vi "P4CMD Get File Copy.vi"(6 "version":string, 8 "error in (no error)":errorcluster, 9 "target filename":path, 10 "source filename":path, 11 "source control reference in":T1) -> (0 "error out":errorcluster, 2 "status message":string, 3 "source control reference out":T1)   [LabVIEW 2020, in "NI_SCC_P4CMD.lvlib"]
uses:
  <vilib>/SourceControl/Providers/P4CMD/NI_SCC_P4CMD.lvlib
  <vilib>/SourceControl/sccapi/SCCAPI Refnum.ctl
  <vilib>/SourceControl/Providers/P4CMD/P4CMD Operations.ctl
  <vilib>/SourceControl/support/SCCSup Message Strings GLBL.vi
  <vilib>/SourceControl/sccapi/NI_SCC.lvlib
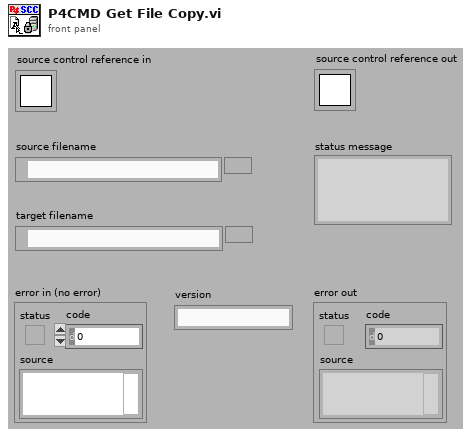
[diagram p1: front panel]
types:
  T1 = typedef "NI_SCC.lvlib/SCCAPI Refnum.ctl" = refnum<k1>
  T2 = typedef "NI_SCC_P4CMD.lvlib/P4CMD Operations.ctl" = enum16{"get all clients", "get all users", "describe changelist", "sync from depot", "open for edit", "submit to depot", "revert", "add to depot", "remove from depot", "print files revisions", "compare client file", "print depot file contents", "list opened files", "get file info", "lock files", "edit changelist spec", "info", "set variables"}
  T3 = typedef "NI_SCC_P4CMD.lvlib/P4CMD SCC File Status.ctl" = cluster{"source controlled":bool, "open by user":bool, "open by other":bool, "out of date":bool, "deleted":bool, "locked by user":bool, "locked by other":bool, "open for add by user":bool, "open for delete by user":bool}
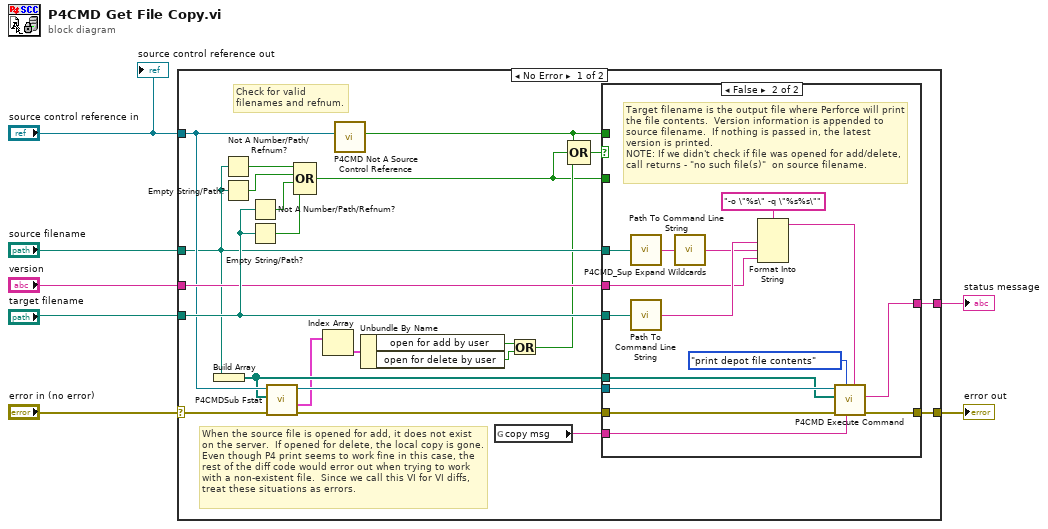
[diagram p0: block diagram]
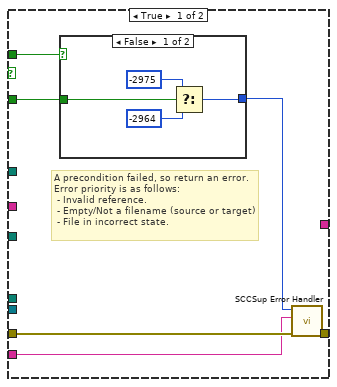
[diagram p2: hidden frame]
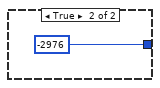
[diagram p3: hidden frame]
diagram:
  n1 = case shown="No Error" "error in (no error)" {
    selector: "error in (no error)" -> [w19 w57]
    tunnel: [w22 w57] -> w6
    tunnel: "source control reference in" -> [w17 _]
    tunnel: [w20 _] -> w4
    tunnel: "source filename" -> [w15 _]
    tunnel: "target filename" -> [w26 _]
    tunnel: "version" -> [w21 _]
    frame No Error {
      # "When the source file is opened for add, it does not exist on the server.  If opened for delete, the local copy is gone.  Even though P4 print seems to work fine in this case, the rest of the diff code would error out when trying to work with a non-existent file.  Since we call this VI for VI diffs, treat these situations as errors."
      # "Check for valid filenames and refnum."
      n2 = Build Array(w15) -> (w14:path[])
      n3 = Not A Number/Path/Refnum?(number/path/refnum=w15) -> (NaN/Path/Refnum?=w29:bool)
      n4 = Empty String/Path?(string/path=w15) -> (empty?=w30:bool)
      n5 = Not A Number/Path/Refnum?(number/path/refnum=w26) -> (NaN/Path/Refnum?=w25:bool)
      n6 = Empty String/Path?(string/path=w26) -> (empty?=w24:bool)
      n7 = call <vilib>:"P4CMDSub Fstat.vi"("error in (no error)"=w19, "files"=w14, "source control reference in"=w17) -> ("error out"=w18:errorcluster, "files status"=w13:T3[], "source control reference out"=w16:T1)  [unwired: 5 in, 1 out]
      n8 = Compound Arithmetic op=OR(w29, w30, w25, w24) -> (w8:bool)
      n9 = Index Array(array=w13) -> (element=w12:T3)  [unwired: 1 in]
      n10 = call <vilib>:"P4CMD Not A Source Control Reference.vi"("source control reference in"=w17) -> ("not a source control reference?"=w27:bool)  [unwired: 9 in, 1 out]
      n11 = Unbundle By Name(w12) -> ("open for add by user"=w11:bool, "open for delete by user"=w10:bool)
      n12 = global read "SCCSup Message Strings GLBL.vi" "copy msg"() -> (w23:string)
      n13 = Or(x=w11, y=w10) -> (x .or. y?=w9:bool)
      n14 = Compound Arithmetic op=OR(w27, w8, w9) -> (w28:bool)
      n15 = case shown="False" w28 {
        tunnel: w15 -> [_ w53]
        tunnel: w26 -> [_ w56]
        tunnel: w27 -> [w31 _]
        tunnel: w18 -> [w36 w46]
        tunnel: w23 -> [w35 w47]
        tunnel: [w33 w54] -> w22
        tunnel: w21 -> [_ w48]
        tunnel: [_ w50] -> w20
        tunnel: w16 -> [_ w45]
        tunnel: w14 -> [_ w44]
        tunnel: w8 -> [w32 _]
        frame True {
          # "A precondition failed, so return an error. \nError priority is as follows:\n - Invalid reference.  \n - Empty/Not a filename (source or target)\n - File in incorrect state."
          n16 = case shown="False" w31 {
            tunnel: [w38 -2976 ("result")] -> w34
            tunnel: w32 -> [w37 _]
            frame False {
              n17 = Select(t=-2975 ("result"), s=w37, f=-2964 ("result")) -> (s? t:f=w38:i32)
            }
            frame True {
            }
          }
          n18 = call <vilib>:"SCCSup Error Handler.vi"("error in (no error)"=w36, "operation message"=w35, "scc error code"=w34) -> ("error out"=w33:errorcluster)  [unwired: 8 in]
        }
        frame False {
          # "Target filename is the output file where Perforce will print the file contents.  Version information is appended to source filename.  If nothing is passed in, the latest version is printed. \nNOTE: If we didn't check if file was opened for add/delete, call returns - \"no such file(s)\"  on source filename."
          n19 = call <vilib>:"Path To Command Line String.vi"("path"=w53) -> ("string"=w43:string)
          n20 = call <vilib>:"Path To Command Line String.vi"("path"=w56) -> ("string"=w49:string)
          n21 = call <vilib>:"P4CMD_Sup Expand Wildcards.vi"("string input"=w43) -> ("string output"=w42:string)  [unwired: 4 in]
          n22 = Format Into String(format string="-o \"%s\" -q \"%s%s\"", w49, w42, w48) -> (resulting string=w51:string)  [unwired: 2 in, 1 out]
          n23 = call <vilib>:"P4CMD Execute Command.vi"("optional operation parameters"=w51, "operation message"=w47, "p4 operation"=P4CMD_Operations."print depot file contents", "error in (no error)"=w46, "files"=w44, "source control reference in"=w45) -> ("error out"=w54:errorcluster, "command information"=w50:string)  [unwired: 3 in, 1 out]
        }
      }
    }
    frame Error {
    }
  }
  "error out" <- w6
  "status message" <- w4
  "source control reference out" <- "source control reference in"
